vi "Condition.vi"(8 "error in":errorcluster, 11 "Msg in":refnum<class "Msg.lvclass">) -> (0 "error out":errorcluster, 3 "Msg out":refnum<class "Msg.lvclass">)   [LabVIEW 2025, in "_Rescript.lvlib" / "Msg.lvlib" / "Msg.lvclass"]
uses:
  Msg.lvclass
  IO.ctl
  Msg.lvclass/Msg.ctl
  _Shared/Name Specs/Name Specs.lvclass
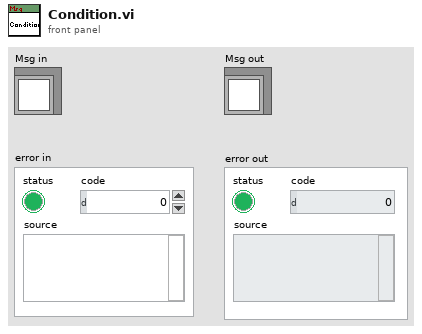
[diagram p1: front panel]
types:
  T1 = typedef "_Rescript.lvlib/Msg.lvlib/Msg.lvclass/IO.ctl" = enum16{"Input", "Output"}
  T2 = typedef "_Rescript.lvlib/Msg.lvlib/Msg.lvclass/Name.ctl" = cluster{"Name VI (Lib)":refnum<vi>, "Init Msg VI (Lib)":refnum<vi>, "Call VI (Lib)":refnum<vi>, "Recurse VI (Lib)":refnum<vi>, "Tell Self VI (Lib)":refnum<vi>, "Tell Parent VI (Lib)":refnum<vi>, "Tell Child VI (Lib)":refnum<vi>, "Tell Reply VI (Lib)":refnum<vi>}
  T3 = typedef "_Rescript.lvlib/Terminals.ctl" = set{i32}
  T4 = typedef "_Rescript.lvlib/Msg.lvlib/Msg.lvclass/Name Msg IO.ctl" = cluster{"PD Control (Class)":refnum<vi>, "PD Cluster (Class)":refnum<vi>, "Init Msg IO VI (Class)":refnum<vi>, "Read Msg IO VI (Class)":refnum<vi>, "Init Msg IO VI (Lib)":refnum<vi>, "Read Msg IO VI (Lib)":refnum<vi>, "Terminal Attributes (Init)":T5, "Terminal Attributes (Read)":T5}
  T5 = typedef "_Rescript.lvlib/Terminal Attributes.ctl" = map{i32, T6}
  T6 = typedef "_Rescript.lvlib/Attributes.ctl" = cluster{"Control":refnum<vi>, "Wire Rule":enum16{"Invalid Wire Rule", "Required", "Recommended", "Optional", "Dynamic Dispatch"}}
  T7 = typedef "_Shared.lvlib/Name Stuff.ctl" = cluster{"Type (Enum)":T8, "Type (String)":string, "Name Library File Path":path, "Name":string, "Name Type":string}
  T8 = typedef "_Shared.lvlib/Type.ctl" = enum16{"Actor", "Msg"}
  T9 = typedef "_Rescript.lvlib/Msg.lvlib/Msg.lvclass/Name Msg.ctl" = cluster{"Execute VI (Class)":refnum<vi>}
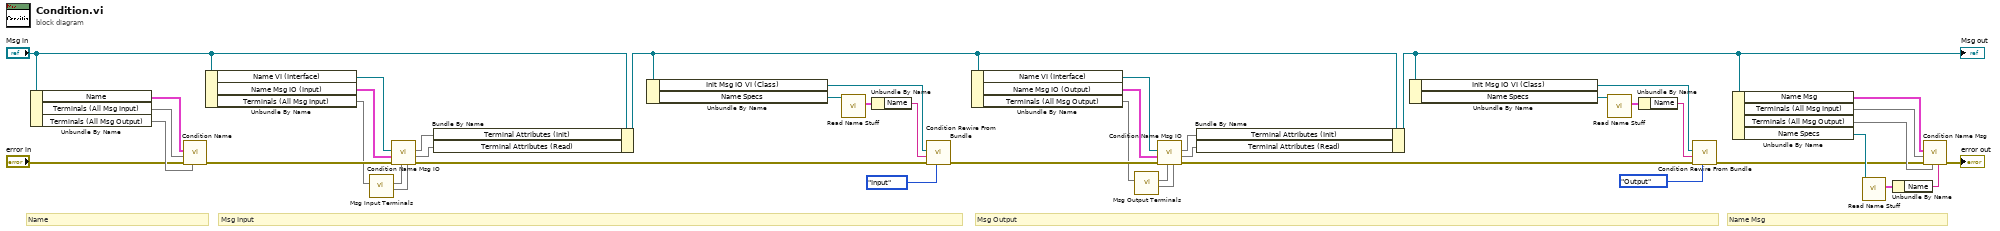
[diagram p0: block diagram]
diagram:
  # "Name Msg"
  # "Msg Output"
  # "Name"
  # "Msg Input"
  n1 = Unbundle By Name("Msg in") -> ("Name"=w42:T2, "Terminals (All Msg Input)"=w41:T3, "Terminals (All Msg Output)"=w40:T3)
  n2 = call "Condition Name.vi"("Terminals (All Msg Output)"=w40, "error in"="error in", "Terminals (All Msg Input)"=w41, "Name"=w42) -> ("error out"=w43:errorcluster)  [unwired: 7 in]
  n3 = Unbundle By Name("Msg in") -> ("Name VI (Interface)"=w35:refnum<vi>, "Name Msg IO (Input)"=w37:T4, "Terminals (All Msg Input)"=w24:T3)
  n4 = call "Msg Input Terminals.vi"("Terminals"=w24) -> ("Terminals (Read Msg Input)"=w26:T3, "Terminals (Init Msg Input)"=w25:T3)  [unwired: 9 in]
  n5 = call "Condition Name Msg IO.vi"("Terminals (All Read)"=w26, "Terminals (All Init)"=w25, "error in"=w43, "Name Msg IO"=w37, "Name jettl Msg.Name VI (Interface)"=w35) -> ("error out"=w19:errorcluster, "Terminal Attributes (Read)"=w28:T5, "Terminal Attributes (Init)"=w27:T5)  [unwired: 4 in]
  n6 = Bundle By Name(cluster="Msg in", "Terminal Attributes (Init)"=w27, "Terminal Attributes (Read)"=w28) -> (w1:refnum<class "Msg.lvclass">)
  n7 = Unbundle By Name(w1) -> ("Init Msg IO VI (Class)"=w20:refnum<vi>, "Name Specs"=w23:refnum<class "Name Specs.lvclass">)
  n8 = call "Read Name Stuff.vi"("Name Specs in"=w23) -> ("Name Stuff"=w22:T7)  [unwired: 10 in]
  n9 = Unbundle By Name(w22) -> ("Name"=w21:string)
  n10 = call "Condition Rewire From Bundle.vi"("IO"=IO."Input", "error in"=w19, "Name"=w21, "VI?"=w20) -> ("error out"=w8:errorcluster)  [unwired: 7 in]
  n11 = Unbundle By Name(w1) -> ("Name VI (Interface)"=w16:refnum<vi>, "Name Msg IO (Output)"=w17:T4, "Terminals (All Msg Output)"=w4:T3)
  n12 = call "Msg Output Terminals.vi"("Terminals (Msg Output)"=w4) -> ("Terminals (Read Msg Output)"=w5:T3, "Terminals (Init Msg Output)"=w6:T3)  [unwired: 9 in]
  n13 = call "Condition Name Msg IO.vi"("Terminals (All Read)"=w5, "Terminals (All Init)"=w6, "error in"=w8, "Name Msg IO"=w17, "Name jettl Msg.Name VI (Interface)"=w16) -> ("error out"=w9:errorcluster, "Terminal Attributes (Read)"=w15:T5, "Terminal Attributes (Init)"=w14:T5)  [unwired: 4 in]
  n14 = Bundle By Name(cluster=w1, "Terminal Attributes (Init)"=w14, "Terminal Attributes (Read)"=w15) -> (w2:refnum<class "Msg.lvclass">)
  "Msg out" <- w2
  n15 = Unbundle By Name(w2) -> ("Init Msg IO VI (Class)"=w10:refnum<vi>, "Name Specs"=w13:refnum<class "Name Specs.lvclass">)
  n16 = call "Read Name Stuff.vi"("Name Specs in"=w13) -> ("Name Stuff"=w12:T7)  [unwired: 10 in]
  n17 = Unbundle By Name(w12) -> ("Name"=w11:string)
  n18 = call "Condition Rewire From Bundle.vi"("IO"=IO."Output", "error in"=w9, "Name"=w11, "VI?"=w10) -> ("error out"=w7:errorcluster)  [unwired: 7 in]
  n19 = Unbundle By Name(w2) -> ("Name Msg"=w32:T9, "Terminals (All Msg Input)"=w29:T3, "Terminals (All Msg Output)"=w30:T3, "Name Specs"=w38:refnum<class "Name Specs.lvclass">)
  n20 = call "Read Name Stuff.vi"("Name Specs in"=w38) -> ("Name Stuff"=w39:T7)  [unwired: 10 in]
  n21 = Unbundle By Name(w39) -> ("Name"=w31:string)
  n22 = call "Condition Name Msg.vi"("Name"=w31, "Terminals (All Msg Output)"=w30, "error in"=w7, "Terminals (All Msg Input)"=w29, "Name Msg"=w32) -> ("error out"=→"error out":errorcluster)  [unwired: 6 in]
